vi "hatchPanelLock.vi"(10 "?":T3=enum."Locked ", 11 "Lock SolenoidDevRef":T1={"DevStatus"={"status"=FALSE, "code"=0, "source"=""}, "Pneumatics Control Module"=0, "Forward Solenoid Channel"=enum."Invalid", "Reverse Solenoid Channel"=enum."Invalid"}) -> ()   [LabVIEW 2018]
uses:
  hatchPanelLockEnum.ctl
  <vilib>/Rock Robotics/WPI/Solenoid/WPI_SolenoidDevRef.ctl
  <vilib>/Rock Robotics/WPI/Solenoid/WPI_SolenoidChannel.ctl
  <vilib>/Rock Robotics/WPI/Solenoid/WPI_SolenoidValue.ctl
  <vilib>/Rock Robotics/WPI/Solenoid/WPI_SolenoidSetEnum.vi
  <userlib>/836-Library/System/TDMS_V2/Support/TDMS_DevRef.ctl
  <userlib>/836-Library/System/TDMS_V2/Support/Logging_Settings.ctl
  <userlib>/836-Library/System/TDMS_V2/Support/Group_FIFO_Config.ctl
  <userlib>/836-Library/System/TDMS_V2/Support/Channel_FIFO_Config.ctl
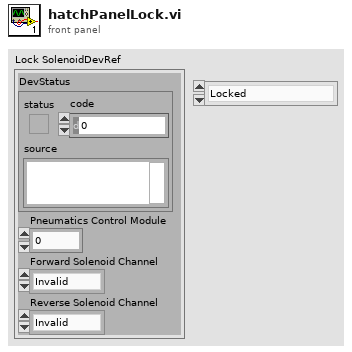
[diagram p1: front panel]
types:
  T1 = typedef "WPI_SolenoidDevRef.ctl" = cluster{"DevStatus":errorcluster, "Pneumatics Control Module":u8, "Forward Solenoid Channel":T2, "Reverse Solenoid Channel":T2}
  T2 = typedef "WPI_SolenoidChannel.ctl" = enum8{"Solenoid 0", "Solenoid 1", "Solenoid 2", "Solenoid 3", "Solenoid 4", "Solenoid 5", "Solenoid 6", "Solenoid 7", "Invalid"}
  T3 = typedef "hatchPanelLockEnum.ctl" = enum16{"Unlocked", "Locked "}
  T4 = typedef "TDMS_DevRef.ctl" = cluster{"Name":string, "File Ref":refnum<k34>, "Start Time":timestamp, "Logging Settings":T5, "Group FIFO Config":T6[], "Data To Write":refnum<data-value>, "semaphore":T8, "Ref Time Reset":refnum<k4>}
  T5 = typedef "Logging_Settings.ctl" = cluster{"Data Grab Period":dbl, "File Write Period":dbl, "Max Stored Size":dbl, "Burst Size":dbl}
  T6 = typedef "Group_FIFO_Config.ctl" = cluster{"Group":string, "Channels":T7[], "Channel Names":string[]}
  T7 = typedef "Channel_FIFO_Config.ctl" = cluster{"Channel":string, "FIFO":refnum<k33>}
  T8 = typedef "Semaphore RefNum" = refnum<k1>
  T9 = typedef "WPI_SolenoidValue.ctl" = enum16{"Off", "On", "Forward", "Reverse"}
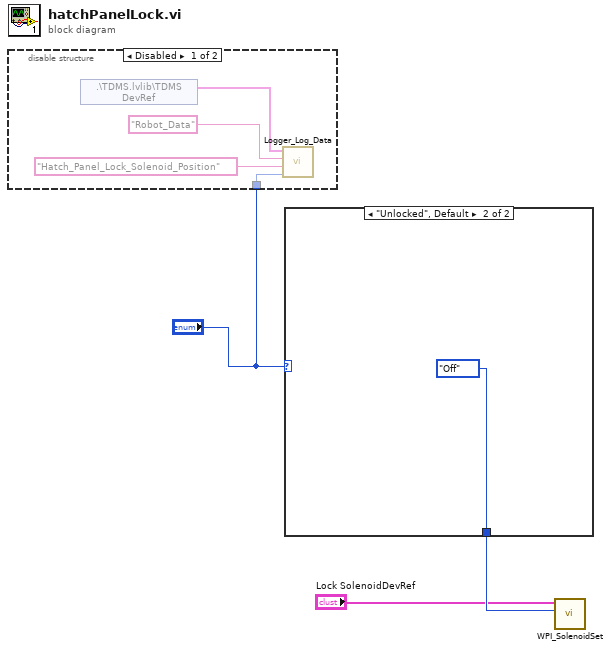
[diagram p0: block diagram]
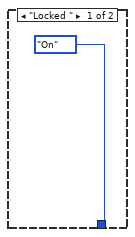
[diagram p3: hidden frame]
diagram:
  n1 = disable-structure shown="Disabled" {
    disable-tunnel: "?" -> [w7 _]
    frame Disabled {
      n2 = shared-variable ".\\TDMS.lvlib\\TDMS DevRef"() -> (w5:T4)  [unwired: 1 in, 1 out]
      n3 = call <userlib>:"Logger_Log_Data.vi"("Data"=w7, "Channel"="Hatch_Panel_Lock_Solenoid_Position", "Group"="Robot_Data", "TDMS DevRef"=w5) -> ()  [unwired: 7 in, 1 out]
    }
    frame Enabled {
    }
  }
  n4 = case shown="\"Unlocked\", Default" "?" {
    tunnel: [WPI_SolenoidValue."On" ("Value") WPI_SolenoidValue."Off" ("Value")] -> w3
    frame "Locked " {
    }
    frame "Unlocked", Default {
    }
  }
  n5 = call-poly <vilib>:"WPI_SolenoidSet.vi"("Value"=w3, "SolenoidDevRef"="Lock SolenoidDevRef") -> ()  [unwired: 8 in, 2 out]
